vi "Numerical Conversion.vi"(1 "SerNmuber":i32, 2 "length":i32) -> (0 "SerNmuber":string)   [LabVIEW 2018]
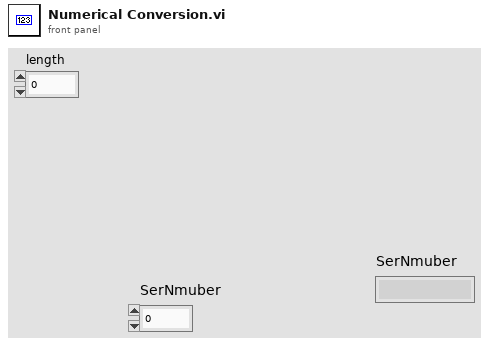
[diagram p1: front panel]
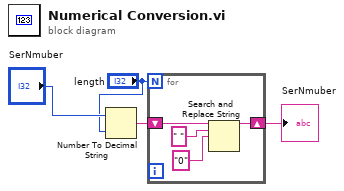
[diagram p0: block diagram]
diagram:
  n1 = Number To Decimal String(number="SerNmuber", width (-)="length") -> (decimal integer string=w4:string)
  n2 = for {
    N: "length" -> [_]
    shift-right: [w5] -> w3
    shift-left: w4 -> [w8]
    n3 = Search and Replace String(input string=w8, search string=" " ("搜索字符串"), replace string="0" ("替换字符串(\"\")")) -> (result string=w5:string)  [unwired: 1 in, 7 out]
  }
  "SerNmuber" <- w3
